vi "Error Query.vi"(7 "Address":u16, 8 "Error in":errorcluster, 11 "VISA Resource in":refnum<visa-resource-name>) -> (0 "Error Out":errorcluster, 1 "Error Message":string, 2 "Error Code":i32[](array[numeric]), 3 "VISA Resource in":refnum<visa-resource-name>)   [LabVIEW 2014, in "KIT QV.lvlib"]
doc: "Queries the instrument for any errors in the instrument's error queue. It will continue to read errors until all errors have been read from the instrument. Any errors will be returned in the <B>error out</B> control.\n\n<B>Note:</B>\nThis VI is called automatically by most driver VIs so it is not usually necessary to call this in an application.\n\n<B>Attention:</B>\nError query is not supported!"
uses:
  KIT QV.lvlib
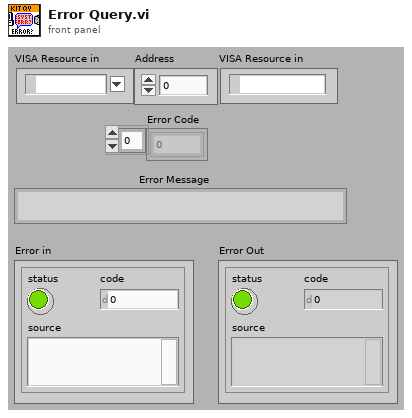
[diagram p1: front panel]
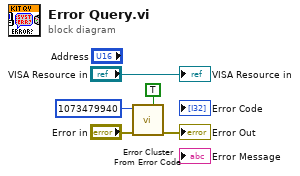
[diagram p0: block diagram]
diagram:
  n1 = call <vilib>:"Error Cluster From Error Code.vi"("is warning? (False)"=TRUE, "error in (no error)"="Error in", "error code (0)"=1073479940) -> ("error out"=→"Error Out":errorcluster)  [unwired: 6 in]
  "VISA Resource in" <- "VISA Resource in"
